vi "Write to TDMS.vi"(8 "error in (no error)":errorcluster, 10 "TDMS File Ref":refnum<k34>, 11 "2D Double Data in":refnum<class "2D Double Logging Data.lvclass">) -> (0 "error out":errorcluster)   [LabVIEW 2024, in "Logging Data.lvlib" / "2D Double Logging Data.lvclass"]
uses:
  2D Double Logging Data.lvclass
  C:/Users/uspoaotto/OneDrive - Oregon Tool/Desktop/working copies/dataLogger/Logging Data/Logging Data/Logging Data.lvclass
  2D Double Logging Data.lvclass/2D Double Logging Data.ctl
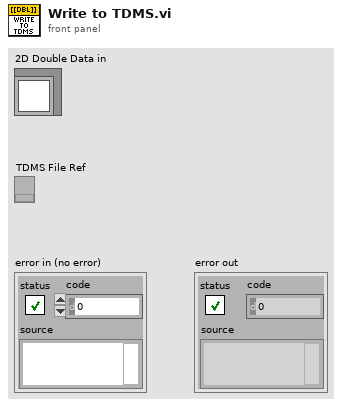
[diagram p1: front panel]
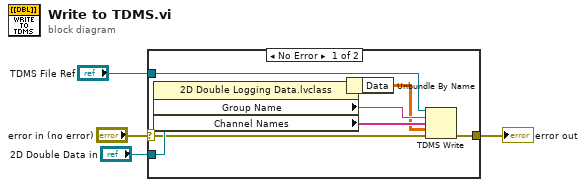
[diagram p0: block diagram]
diagram:
  n1 = case shown="No Error" "error in (no error)" {
    selector: "error in (no error)" -> [w6 w13]
    tunnel: "2D Double Data in" -> [w12 _]
    tunnel: "TDMS File Ref" -> [w7 _]
    tunnel: [w5 w13] -> w1
    frame No Error {
      n2 = property class="2D Double Logging Data.lvclass"(reference=w12) -> (reference out=w9:refnum<class "2D Double Logging Data.lvclass">, "Group Name"=w11:string, "Channel Names"=w10:string[])  [unwired: 1 in, 1 out]
      n3 = Unbundle By Name(w9) -> ("Data"=w8:dbl[][])
      n4 = TDMS Write(0:w7, 5:w11, 7:w10, 9:w8, 11:w6) -> (15:w5:errorcluster)  [unwired: 1 in, 3 out]
    }
    frame Error {
    }
  }
  "error out" <- w1
